vi "CalibrationTool.vi"() -> ()   [LabVIEW 2018]
uses:
  <vilib>/userdefined/High Color/IMAQdx.ctl
  <vilib>/vision/driver/NI_Vision_Acquisition_Software.lvlib
panel:
  in  "stop":bool
  out "Image Out":T1(plugin-control)
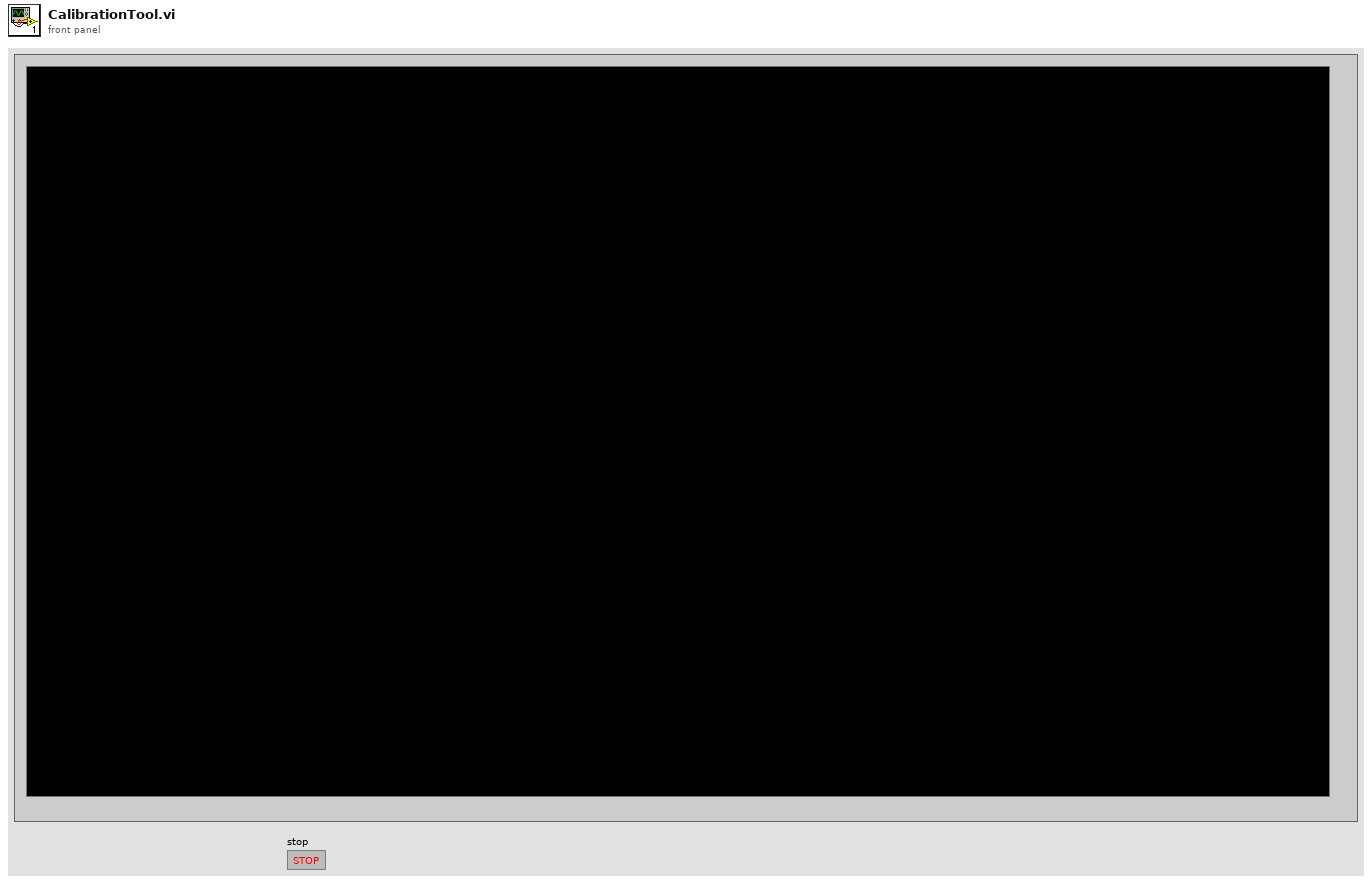
[diagram p1: front panel]
types:
  T1 = typedef "IMAQ Image.ctl" = refnum<image>
  T2 = typedef "Image Type" = u32
  T3 = typedef "IMAQdx.ctl" = refnum<k21>
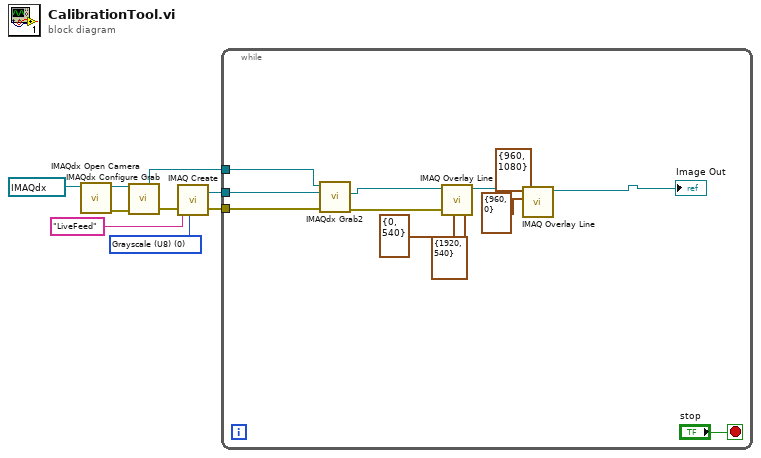
[diagram p0: block diagram]
diagram:
  w4 = T2 0 items=["Grayscale (U8)", "Grayscale (I16)", "Grayscale (SGL)", "Complex (CSG)", "RGB (U32)", "HSL (U32)", "RGB (U64)", "Grayscale (U16)"] ("Image Type")
  n1 = call <vilib>:"IMAQdx Open Camera.vi"("Session In"=T3 "cam0") -> ("error out"=w7:errorcluster, "Session Out"=w8:T3)  [unwired: 9 in]
  n2 = call <vilib>:"IMAQdx Configure Grab.vi"("error in"=w7, "Session In"=w8) -> ("error out"=w5:errorcluster, "Session Out"=w3:T3)  [unwired: 8 in]
  n3 = call "IMAQ Create"("Image Name"="LiveFeed", "Image Type"=w4, "error in (no error)"=w5) -> ("New Image"=w2:T1, "error out"=w1:errorcluster)  [unwired: 2 in]
  n4 = while {
    tunnel: w3 -> [w21]
    tunnel: w2 -> [w20]
    tunnel: w1 -> [w19]
    stop <- "stop" stop-if-true
    n5 = call <vilib>:"IMAQdx Grab2.vi"("error in"=w19, "Image In"=w20, "Session In"=w21) -> ("error out"=w15:errorcluster, "Image Out"=w16:T1)  [unwired: 5 in, 2 out]
    n6 = call "IMAQ Overlay Line"("error in (no error)"=w15, "End Point"=cluster{"X":i32, "Y":i32} {"X"=1920, "Y"=540}, "Start Point"=cluster{"X":i32, "Y":i32} {"X"=0, "Y"=540}, "Image"=w16) -> ("Image Out"=w14:T1)  [unwired: 6 in, 1 out]
    n7 = call "IMAQ Overlay Line"("End Point"=cluster{"X":i32, "Y":i32} {"X"=960, "Y"=1080}, "Start Point"=cluster{"X":i32, "Y":i32} {"X"=960, "Y"=0}, "Image"=w14) -> ("Image Out"=→"Image Out":T1)  [unwired: 7 in, 1 out]
  }
